vi "Generator.Create Reference Waveforms.vi"(8 "error in (no error)":errorcluster, 10 "reset phase":bool, 11 "Generator in":refnum<class "Generator.lvclass">) -> (0 "error out":errorcluster, 1 "Y":waveform(dbl)[](array[waveform]), 2 "X":waveform(dbl)[](array[waveform]), 3 "Generator out":refnum<class "Generator.lvclass">, 6 "sampling info":cluster{"Fs":dbl, "#s":dbl}={"Fs"=1000.0, "#s"=1000.0} {"Fs" format="%.2p"})   [LabVIEW 2019, in "Generator.lvclass"]
uses:
  Generator.lvclass
  <vilib>/measure/NI_MABase.lvlib
  Instrument.DAQ/Instrument.DAQ.lvclass
  Instrument.DAQ/Typedefs/REF.Channel--Cluster.ctl
  Instrument.DAQ/Typedefs/REF.Channel--Cluster--Array.ctl
panel:
  in  "Tab Control":enum32{"Page 1", "Graph"}(tab)
  out "Configuration.Channels: REF":T1 {"Roll-Off" min=1; "TC" min=0.0001 format="%#_3p"; "Phase" format="%.3g"; "Frequency" min=0.0001 max=10000.0 format="%.3g"; "Channel" min=1}
  out "Waveform Graph":waveform(dbl)[](graph)
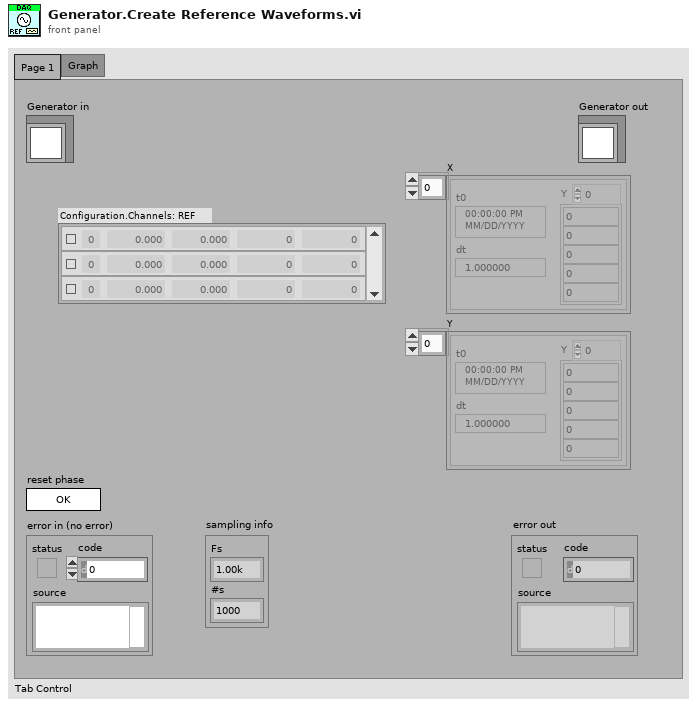
[diagram p1: front panel]
types:
  T1 = typedef "Instrument.Lockin.lvlib/Instrument.DAQ.lvclass/REF.Channel--Cluster--Array.ctl" = T2[]
  T2 = typedef "Instrument.Lockin.lvlib/Instrument.DAQ.lvclass/REF.Channel--Cluster.ctl" = cluster{"Enable?":bool, "Channel":i32, "Frequency":dbl, "Phase":dbl, "TC":dbl, "Roll-Off":i32}
  T3 = enum16{"Sine Wave", "Triangle Wave", "Square Wave", "Sawtooth Wave"}
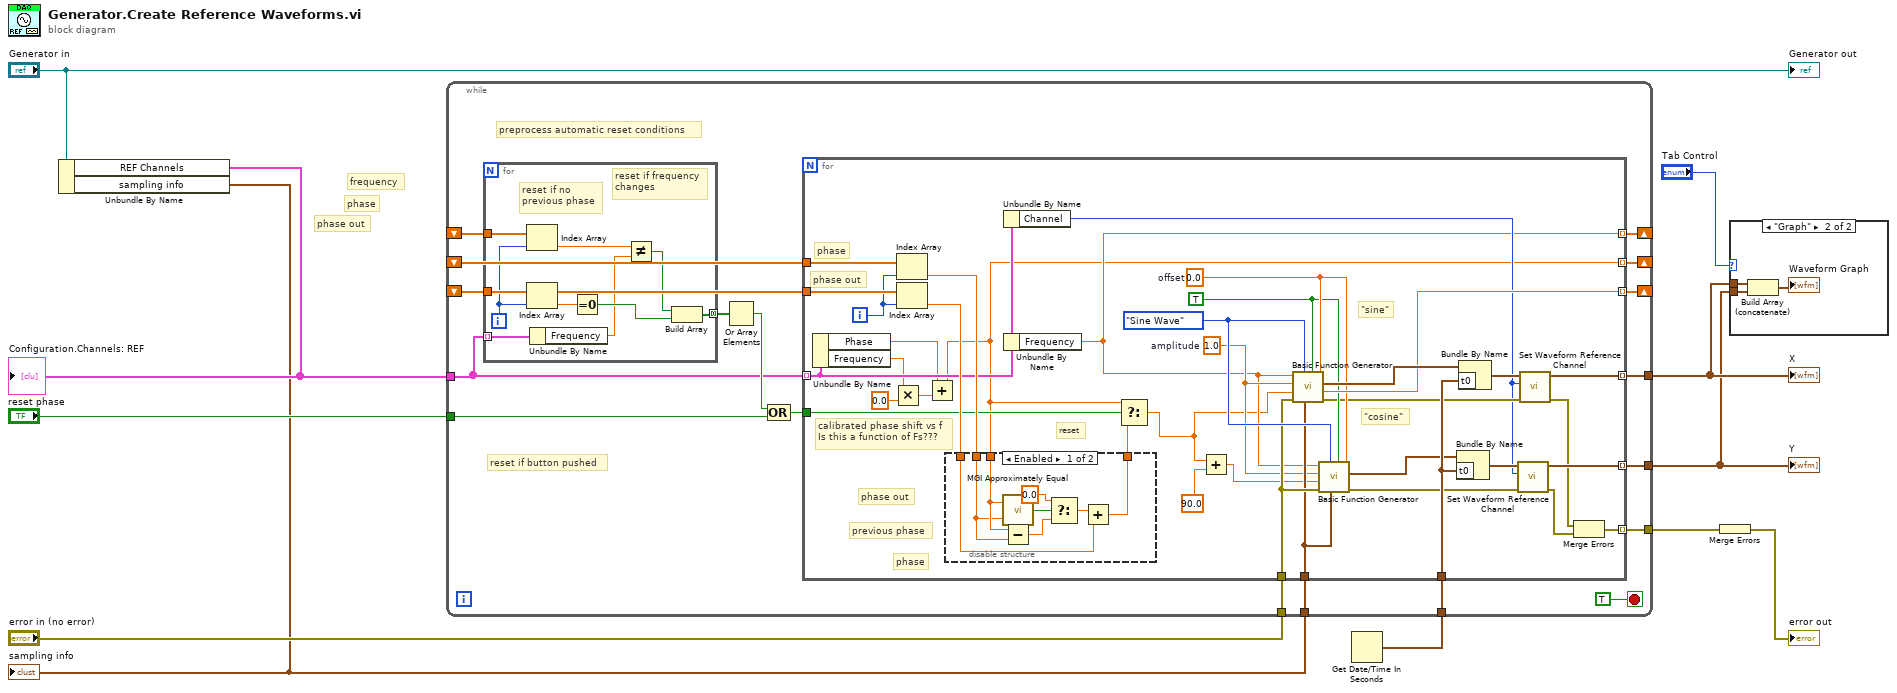
[diagram p0: block diagram]
diagram:
  # "phase out"
  # "phase"
  # "frequency"
  n1 = Unbundle By Name("Generator in") -> ("REF Channels"=w2:T1, "sampling info"=w1:cluster{"Fs":dbl, "#s":dbl})
  "sampling info" <- w1
  "Configuration.Channels: REF" <- w2
  n2 = Get Date/Time In Seconds() -> (seconds since 1Jan1904=w10:timestamp)
  n3 = while {
    tunnel: w1 -> [w29]
    shift-right: [w27] -> _
    shift-left: _ -> [w21]
    tunnel: w10 -> [w26]
    tunnel: "reset phase" -> [w16]
    tunnel: "error in (no error)" -> [w25]
    tunnel: w2 -> [w14]
    shift-right: [w24] -> _
    shift-left: _ -> [w19]
    shift-right: [w23] -> _
    shift-left: _ -> [w20]
    tunnel: [w22] -> w8
    tunnel: [w13] -> w7
    tunnel: [w12] -> w6
    stop <- TRUE stop-if-true
    # "preprocess automatic reset conditions"
    # "reset if button pushed"
    n4 = for {
      tunnel: w14 -> [w31] mode=indexing
      tunnel: w21 -> [w38]
      tunnel: w19 -> [w37]
      tunnel: [w32] -> w18 mode=concatenating
      i -> [w39]
      # "reset if frequency\nchanges"
      # "reset if no\nprevious phase"
      n5 = Index Array(array=w37, index=w39) -> (element=w35:dbl)
      n6 = Index Array(array=w38, index=w39) -> (element=w36:dbl)
      n7 = Unbundle By Name(w31) -> ("Frequency"=w30:dbl)
      n8 = Equal To 0?(x=w36) -> (x = 0?=w33:bool)
      n9 = Not Equal?(x=w35, y=w30) -> (x != y?=w34:bool)
      n10 = Build Array(w34, w33) -> (w32:bool[])
    }
    n11 = Or Array Elements(Boolean array=w18) -> (logical OR=w17:bool)
    n12 = Compound Arithmetic op=OR(w17, w16) -> (w15:bool)
    n13 = for {
      tunnel: w29 -> [w68]
      tunnel: [w74] -> w27 mode=indexing
      tunnel: w26 -> [w73]
      tunnel: w25 -> [w69]
      tunnel: w14 -> [w49] mode=indexing
      tunnel: w21 -> [w65]
      tunnel: [w46] -> w24 mode=indexing
      tunnel: [w40] -> w23 mode=indexing
      tunnel: w15 -> [w59]
      tunnel: w20 -> [w64]
      tunnel: [w63] -> w22 mode=indexing
      tunnel: [w57] -> w13 mode=indexing
      tunnel: [w55] -> w12 mode=indexing
      i -> [w54]
      w66 = TRUE ("reset signal")
      w70 = 0.0  # offset
      w71 = T3."Sine Wave" ("signal type")
      w67 = 1.0  # amplitude
      # "calibrated phase shift vs f\nIs this a function of Fs???"
      # "phase out"
      # "phase"
      # "previous phase"
      # "phase"
      # "phase out"
      # "reset"
      # "\"cosine\""
      # "\"sine\""
      n14 = Unbundle By Name(w49) -> ("Phase"=w41:dbl, "Frequency"=w43:dbl)
      n15 = Multiply(x=w43, y=0.0) -> (x*y=w42:dbl)
      n16 = Index Array(array=w64, index=w54) -> (element=w62:dbl)
      n17 = Index Array(array=w65, index=w54) -> (element=w60:dbl)
      n18 = Add(x=w41, y=w42) -> (x+y=w40:dbl)
      n19 = disable-structure shown="Enabled" {
        disable-tunnel: w40 -> [w83 _]
        disable-tunnel: w62 -> [w82 _]
        disable-tunnel: w60 -> [w77 w85]
        disable-tunnel: [w80 w85] -> w61
        frame Enabled {
          n20 = call <userlib>:"MGI Approximately Equal.vi"("Numeric 2"=w82, "Numeric 1"=w83) -> ("approx = ?"=w81:bool)
          n21 = Subtract(x=w83, y=w82) -> (x-y=w79:dbl)
          n22 = Select(t=0.0, s=w81, f=w79) -> (s? t:f=w78:dbl)
          n23 = Add(x=w78, y=w77) -> (x+y=w80:dbl)
        }
        frame Disabled {
        }
      }
      n24 = Unbundle By Name(w49) -> ("Channel"=w48:i32)
      n25 = Unbundle By Name(w49) -> ("Frequency"=w46:dbl)
      n26 = Select(t=w40, s=w59, f=w61) -> (s? t:f=w44:dbl)
      n27 = Add(x=w44, y=90.0) -> (x+y=w47:dbl)
      n28 = call <vilib>:"Basic Function Generator.vi"("offset"=w70, "reset signal"=w66, "sampling info"=w68, "signal type"=w71, "error in (no error)"=w69, "phase"=w44, "amplitude"=w67, "frequency"=w46) -> ("error out"=w53:errorcluster, "phase out"=w74:dbl, "signal out"=w76:waveform(dbl))  [unwired: 1 in]
      n29 = call <vilib>:"Basic Function Generator.vi"("offset"=w70, "reset signal"=w66, "sampling info"=w68, "signal type"=w71, "error in (no error)"=w69, "phase"=w47, "amplitude"=w67, "frequency"=w46) -> ("error out"=w52:errorcluster, "signal out"=w72:waveform(dbl))  [unwired: 1 in, 1 out]
      n30 = Bundle By Name(cluster=w72, "t0"=w73) -> (w56:waveform(dbl))
      n31 = Bundle By Name(cluster=w76, "t0"=w73) -> (w58:waveform(dbl))
      n32 = call "Set Waveform Reference Channel.vi"("error in (no error)"=w52, "Reference Ch"=w48, "Waveform in"=w56) -> ("error out"=w51:errorcluster, "Waveform out"=w55:waveform(dbl))  [unwired: 7 in]
      n33 = call "Set Waveform Reference Channel.vi"("error in (no error)"=w53, "Reference Ch"=w48, "Waveform in"=w58) -> ("error out"=w50:errorcluster, "Waveform out"=w57:waveform(dbl))  [unwired: 7 in]
      n34 = Merge Errors(w50, w51) -> (w63:errorcluster)
    }
  }
  "X" <- w7
  "Y" <- w6
  n35 = Merge Errors(w8) -> (→"error out":errorcluster)
  n36 = case shown="\"Graph\"" "Tab Control" {
    tunnel: w7 -> [_ w87]
    tunnel: w6 -> [_ w86]
    frame Default {
    }
    frame "Graph" {
      n37 = Build Array (concatenate)(w87, w86) -> (→"Waveform Graph":waveform(dbl)[])
    }
  }
  "Generator out" <- "Generator in"
